vi "Save Color User Items.vi"(6 "save settings?":bool=TRUE, 8 "error in":errorcluster, 9 "Color Names":string[](array[string])=["primary", "onPrimary", "secondary", "onSecondary", "tertiary", "onTertiary", "error", "onError", "surface", "onSurface", "SurfaceVariant"], 10 "colors":u32[](array[colorbox])) -> (0 "error out":errorcluster)   [LabVIEW 2021, in "TSC Material Theme.lvlib" / "Material-Scheme.lvclass"]
doc: "Save out custom colors from the scheme to the <i>colorUserItem</i> tag in the LabVIEW ini file.\n\n<b>Code Developed By:</b>\nDaniel Coons\nTechnology Service Corporation\nwww.tsc.com/atcs"
uses:
  Material-Scheme.lvclass
  Material-Scheme.lvclass/Material-Scheme.ctl
  <resource>/dialog/lvconfig.llb/LV Config Write String.vi
panel:
  out "size(s)":i32
  out "spreadsheet string":string
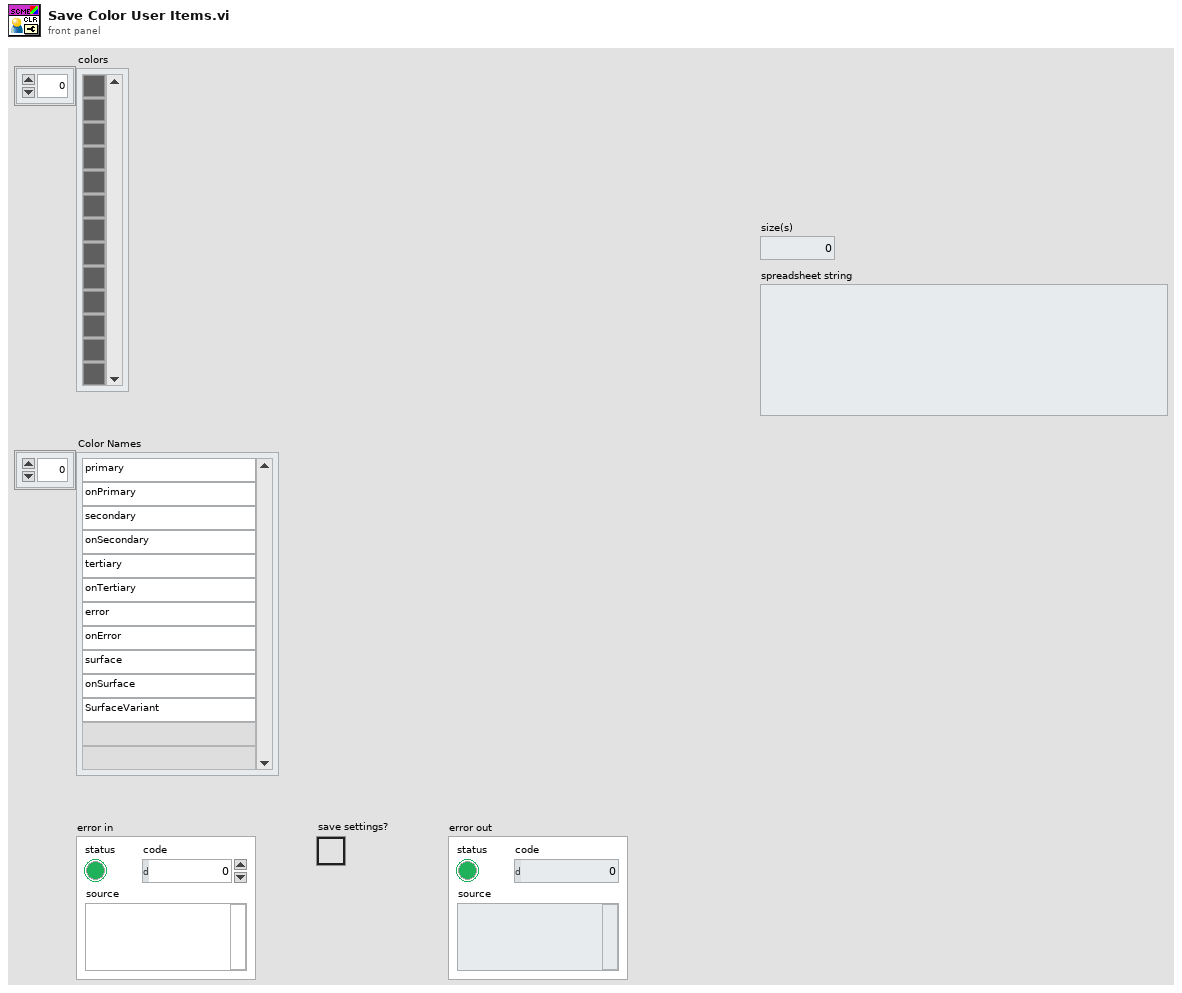
[diagram p1: front panel]
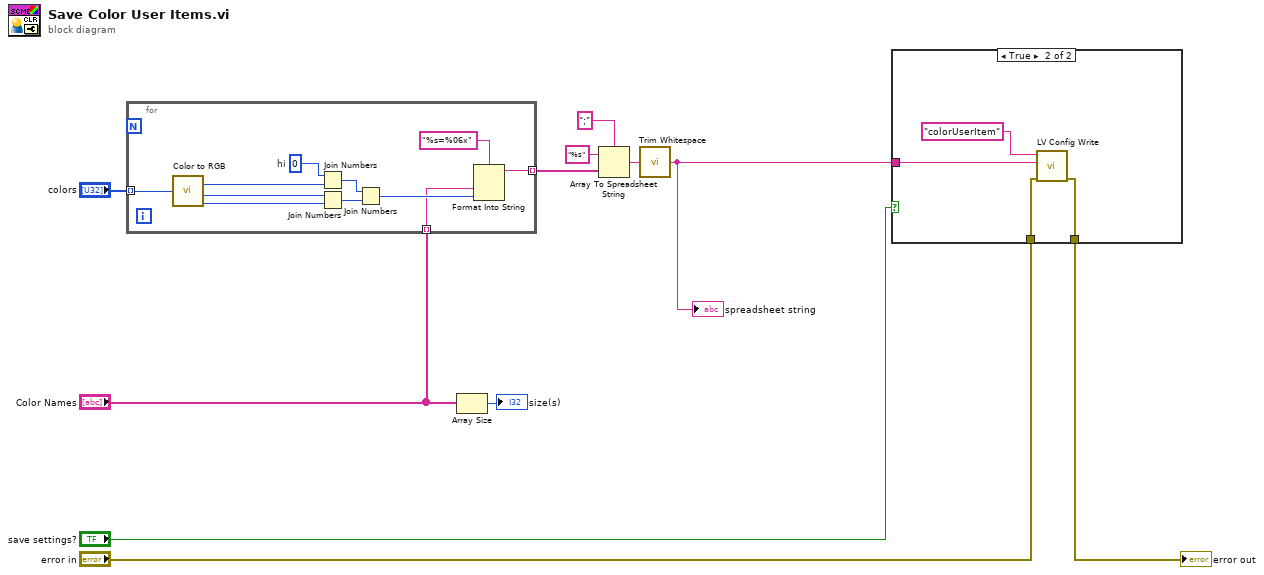
[diagram p0: block diagram]
diagram:
  n1 = for {
    tunnel: "colors" -> [w19] mode=indexing
    tunnel: [w14] -> w11 mode=indexing
    tunnel: "Color Names" -> [w12] mode=indexing
    w22 = u8 0  # hi
    n2 = call <vilib>:"Color to RGB.vi"("Color"=w19) -> ("R"=w17:u8, "G"=w16:u8, "B"=w15:u8)  [unwired: 1 out]
    n3 = Join Numbers(hi=w22, lo=w17) -> ((hi.lo)=w20:u16)
    n4 = Join Numbers(hi=w16, lo=w15) -> ((hi.lo)=w21:u16)
    n5 = Join Numbers(hi=w20, lo=w21) -> ((hi.lo)=w13:u32)
    n6 = Format Into String(format string="%s=%06x", w12, w13) -> (resulting string=w14:string)  [unwired: 2 in, 1 out]
  }
  n7 = Array Size(array="Color Names") -> (size(s)=→"size(s)":i32)
  n8 = Array To Spreadsheet String(delimiter (Tab)=";", array=w11, 3:"%s" ("format string")) -> (spreadsheet string=w8:string)
  n9 = call <vilib>:"Trim Whitespace.vi"("string"=w8) -> ("trimmed string"=w3:string)  [unwired: 1 in]
  "spreadsheet string" <- w3
  n10 = case shown="True" "save settings?" {
    tunnel: "error in" -> [w23 w26]
    tunnel: [w23 w25] -> w4
    tunnel: w3 -> [_ w24]
    frame False {
    }
    frame True {
      n11 = call-poly <resource>:"LV Config Write.vi"("error in (no error)"=w26, "value"=w24, "key"="colorUserItem") -> ("error out"=w25:errorcluster)  [unwired: 4 in]
    }
  }
  "error out" <- w4
